vi "GetFreqOffset.vi"(8 "Error In":errorcluster, 9 "Resp Timeout (ms)":i32 min=0, 10 "Enum":T1, 11 "FPGA Reference":refnum<k20>) -> (0 "Error Out":errorcluster, 1 "Freq Offset (Hz)":ext, 2 "Get Freq Offset OK":bool, 3 "Received Text":string)   [LabVIEW 2018]
uses:
  Resources_Test/UART/ControlTestSlot.ctl
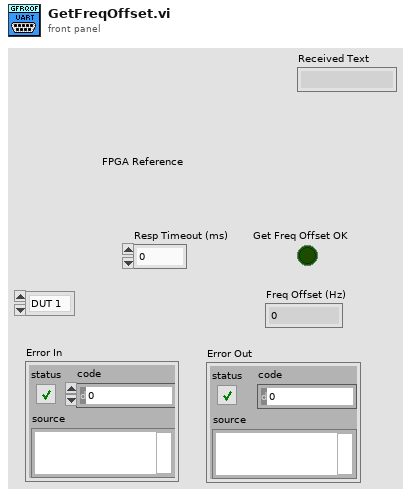
[diagram p1: front panel]
types:
  T1 = typedef "ControlTestSlot.ctl" = enum16{"DUT 1", "DUT 2"}
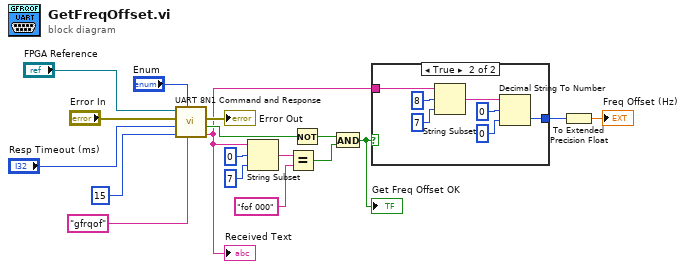
[diagram p0: block diagram]
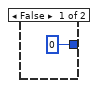
[diagram p2: hidden frame]
diagram:
  n1 = call "UART 8N1 Command and Response.vi"("Text to Send"="gfrqof", "Active Dut"="Enum", "Response Size (char)"=u32 15, "Response Timeout (ms)"="Resp Timeout (ms)", "Error In"="Error In", "FPGA VI Reference In"="FPGA Reference") -> ("Received Text"=w3:string, "Timeout Flag"=w5:bool, "Error Out"=→"Error Out":errorcluster)  [unwired: 2 in, 1 out]
  "Received Text" <- w3
  n2 = String Subset(string=w3, offset (0)=0, length (rest)=7 ("length (rest)")) -> (substring=w13:string)
  n3 = Equal?(x=w13, y="fof 000") -> (x = y?=w17:bool)
  n4 = Not(x=w5) -> (.not. x?=w18:bool)
  n5 = And(x=w18, y=w17) -> (x .and. y?=w4:bool)
  "Get Freq Offset OK" <- w4
  n6 = case shown="True" w4 {
    tunnel: w3 -> [_ w21]
    tunnel: [0 w20] -> w2
    frame False {
    }
    frame True {
      n7 = String Subset(string=w21, offset (0)=8, length (rest)=7 ("length (rest)")) -> (substring=w26:string)
      n8 = Decimal String To Number(string=w26, offset=0, default (0L)=0 ("default (0 I32)")) -> (number=w20:i32)  [unwired: 1 out]
    }
  }
  n9 = To Extended Precision Float(1:w2) -> (0:→"Freq Offset (Hz)":ext)
